vi "BefVibrationStrView.vi"(8 "error in":errorcluster caption="错误输入", 9 "StrIn":string, 10 "Value":variant, 11 "总结果显示":refnum<vi>) -> (0 "error out":errorcluster caption="错误输出", 3 "StrOut":string)   [LabVIEW 2013]
uses:
  Ctl/SinResult.ctl
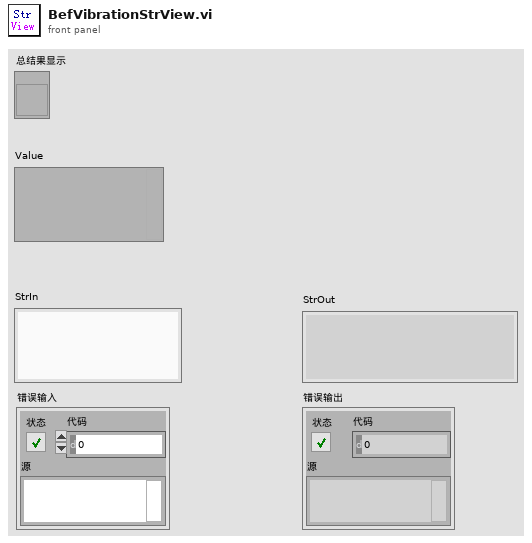
[diagram p1: front panel]
types:
  T1 = typedef "SinResult.ctl" = cluster{"CAN通道":string, "TsRes":bool}
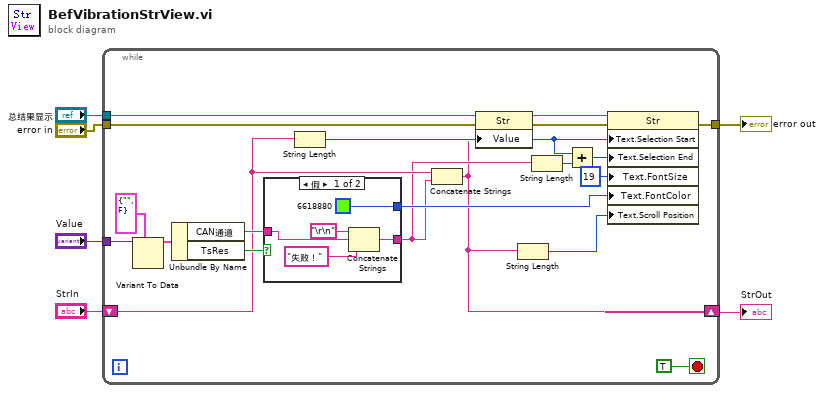
[diagram p0: block diagram]
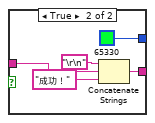
[diagram p2: hidden frame]
diagram:
  n1 = while {
    tunnel: "总结果显示" -> [w25]
    tunnel: "Value" -> [w23]
    tunnel: [w19] -> w4
    tunnel: "error in" -> [w18]
    shift-right: [w7] -> w1
    shift-left: "StrIn" -> [w10]
    stop <- TRUE stop-if-true
    n2 = Variant To Data(type=T1 {"CAN通道"="", "TsRes"=FALSE} ("CAN结果"), Variant=w23) -> (data=w22:T1)  [unwired: 1 in, 1 out]
    n3 = Unbundle By Name(w22) -> ("CAN通道"=w21:string, "TsRes"=w20:bool)
    n4 = case shown="假" w20 {
      tunnel: w21 -> [w28 w33]
      tunnel: [u32 6618880 u32 65330] -> w12
      tunnel: [w29 w34] -> w9
      frame False {
        n5 = Concatenate Strings("\r\n" ("字符串"), w28, "失败！") -> (w29:string)
      }
      frame True {
        n6 = Concatenate Strings("\r\n", w33, "成功！") -> (w34:string)
      }
    }
    n7 = String Length(string=w10) -> (length=w15:i32)
    n8 = Concatenate Strings(w10, w9) -> (w7:string)
    n9 = property class="Str"(reference=w25, "Value"=w7) -> (reference out=w11:refnum<vi>)  [unwired: 1 in, 1 out]
    n10 = String Length(string=w7) -> (length=w8:i32)
    n11 = String Length(string=w9) -> (length=w16:i32)
    n12 = Add(x=w15, y=w16) -> (x+y=w14:i32)
    n13 = property class="Str"(reference=w11, error in=w18, "Text.Selection Start"=w15, "Text.Selection End"=w14, "Text.FontSize"=u32 19 ("文本.字体:字号"), "Text.FontColor"=w12, "Text.Scroll Position"=w8) -> (error out=w19:errorcluster)  [unwired: 1 out]
  }
  "error out" <- w4
  "StrOut" <- w1
